vi "十八仔.vi"() -> ()   [LabVIEW 2014]
panel:
  in  "Listbox 2":i32[](listbox)
  in  "Listbox 3":i32[](listbox)
  in  "Listbox":i32[](listbox)
  in  "遊戲開始":bool
  out "總共賺取/賠掉金額":i32
  out "經歷輪數":i32
  out "此輪賺取/賠掉金額":i32
  out "賭金金額":i32
  in  "Cluster 48":T1={"Color Box 4"=16448250, "Boolean 5"=FALSE, "Boolean 11"=FALSE, "Boolean 12"=FALSE, "Boolean 13"=FALSE, "Boolean 14"=FALSE, "Boolean 15"=FALSE}
  in  "Cluster 47":T2={"Color Box 2"=16777215, "Boolean"=FALSE, "Boolean 3"=FALSE, "Boolean 2"=FALSE}
  in  "Cluster 46":T3={"Color Box"=16777215, "Boolean"=FALSE, "Boolean 2"=FALSE}
  in  "Cluster 45":T4={"Color Box"=16777215, "Boolean"=FALSE}
  in  "Cluster 44":T5={"Color Box"=16777215, "Boolean 4"=FALSE, "Boolean 5"=FALSE, "Boolean 6"=FALSE, "Boolean 7"=FALSE, "Boolean 8"=FALSE}
  in  "Cluster 43":T6={"Color Box 2"=16777215, "Boolean 3"=FALSE, "Boolean 4"=FALSE, "Boolean 6"=FALSE, "Boolean 5"=FALSE}
  in  "Cluster 42":T1={"Color Box 4"=16448250, "Boolean 5"=FALSE, "Boolean 11"=FALSE, "Boolean 12"=FALSE, "Boolean 13"=FALSE, "Boolean 14"=FALSE, "Boolean 15"=FALSE}
  in  "Cluster 41":T2={"Color Box 2"=16777215, "Boolean"=FALSE, "Boolean 3"=FALSE, "Boolean 2"=FALSE}
  in  "Cluster 40":T3={"Color Box"=16777215, "Boolean"=FALSE, "Boolean 2"=FALSE}
  in  "Cluster 39":T4={"Color Box"=16777215, "Boolean"=FALSE}
  in  "Cluster 38":T5={"Color Box"=16777215, "Boolean 4"=FALSE, "Boolean 5"=FALSE, "Boolean 6"=FALSE, "Boolean 7"=FALSE, "Boolean 8"=FALSE}
  in  "Cluster 37":T6={"Color Box 2"=16777215, "Boolean 3"=FALSE, "Boolean 4"=FALSE, "Boolean 6"=FALSE, "Boolean 5"=FALSE}
  in  "Cluster 36":T5={"Color Box"=16777215, "Boolean 4"=FALSE, "Boolean 5"=FALSE, "Boolean 6"=FALSE, "Boolean 7"=FALSE, "Boolean 8"=FALSE}
  in  "Cluster 35":T6={"Color Box 2"=16777215, "Boolean 3"=FALSE, "Boolean 4"=FALSE, "Boolean 6"=FALSE, "Boolean 5"=FALSE}
  in  "Cluster 34":T1={"Color Box 4"=16448250, "Boolean 5"=FALSE, "Boolean 11"=FALSE, "Boolean 12"=FALSE, "Boolean 13"=FALSE, "Boolean 14"=FALSE, "Boolean 15"=FALSE}
  in  "Cluster 33":T2={"Color Box 2"=16777215, "Boolean"=FALSE, "Boolean 3"=FALSE, "Boolean 2"=FALSE}
  in  "Cluster 32":T3={"Color Box"=16777215, "Boolean"=FALSE, "Boolean 2"=FALSE}
  in  "Cluster 31":T4={"Color Box"=16777215, "Boolean"=FALSE}
  in  "Cluster 30":T1={"Color Box 4"=16448250, "Boolean 5"=FALSE, "Boolean 11"=FALSE, "Boolean 12"=FALSE, "Boolean 13"=FALSE, "Boolean 14"=FALSE, "Boolean 15"=FALSE}
  in  "Cluster 29":T2={"Color Box 2"=16777215, "Boolean"=FALSE, "Boolean 3"=FALSE, "Boolean 2"=FALSE}
  in  "Cluster 28":T3={"Color Box"=16777215, "Boolean"=FALSE, "Boolean 2"=FALSE}
  in  "Cluster 27":T4={"Color Box"=16777215, "Boolean"=FALSE}
  in  "Cluster 26":T5={"Color Box"=16777215, "Boolean 4"=FALSE, "Boolean 5"=FALSE, "Boolean 6"=FALSE, "Boolean 7"=FALSE, "Boolean 8"=FALSE}
  in  "Cluster 25":T6={"Color Box 2"=16777215, "Boolean 3"=FALSE, "Boolean 4"=FALSE, "Boolean 6"=FALSE, "Boolean 5"=FALSE}
  in  "Cluster 24":T5={"Color Box"=16777215, "Boolean 4"=FALSE, "Boolean 5"=FALSE, "Boolean 6"=FALSE, "Boolean 7"=FALSE, "Boolean 8"=FALSE}
  in  "Cluster 23":T6={"Color Box 2"=16777215, "Boolean 3"=FALSE, "Boolean 4"=FALSE, "Boolean 6"=FALSE, "Boolean 5"=FALSE}
  in  "Cluster 22":T1={"Color Box 4"=16448250, "Boolean 5"=FALSE, "Boolean 11"=FALSE, "Boolean 12"=FALSE, "Boolean 13"=FALSE, "Boolean 14"=FALSE, "Boolean 15"=FALSE}
  in  "Cluster 21":T2={"Color Box 2"=16777215, "Boolean"=FALSE, "Boolean 3"=FALSE, "Boolean 2"=FALSE}
  in  "Cluster 20":T3={"Color Box"=16777215, "Boolean"=FALSE, "Boolean 2"=FALSE}
  in  "Cluster 19":T4={"Color Box"=16777215, "Boolean"=FALSE}
  in  "Cluster 18":T3={"Color Box"=16777215, "Boolean"=FALSE, "Boolean 2"=FALSE}
  in  "Cluster 17":T4={"Color Box"=16777215, "Boolean"=FALSE}
  in  "Cluster 16":T5={"Color Box"=16777215, "Boolean 4"=FALSE, "Boolean 5"=FALSE, "Boolean 6"=FALSE, "Boolean 7"=FALSE, "Boolean 8"=FALSE}
  in  "Cluster 15":T6={"Color Box 2"=16777215, "Boolean 3"=FALSE, "Boolean 4"=FALSE, "Boolean 6"=FALSE, "Boolean 5"=FALSE}
  in  "Cluster 14":T1={"Color Box 4"=16448250, "Boolean 5"=FALSE, "Boolean 11"=FALSE, "Boolean 12"=FALSE, "Boolean 13"=FALSE, "Boolean 14"=FALSE, "Boolean 15"=FALSE}
  in  "Cluster 13":T2={"Color Box 2"=16777215, "Boolean"=FALSE, "Boolean 3"=FALSE, "Boolean 2"=FALSE}
  in  "Cluster 12":T5={"Color Box"=16777215, "Boolean 4"=FALSE, "Boolean 5"=FALSE, "Boolean 6"=FALSE, "Boolean 7"=FALSE, "Boolean 8"=FALSE}
  in  "Cluster 11":T6={"Color Box 2"=16777215, "Boolean 3"=FALSE, "Boolean 4"=FALSE, "Boolean 6"=FALSE, "Boolean 5"=FALSE}
  in  "Cluster 10":T1={"Color Box 4"=16448250, "Boolean 5"=FALSE, "Boolean 11"=FALSE, "Boolean 12"=FALSE, "Boolean 13"=FALSE, "Boolean 14"=FALSE, "Boolean 15"=FALSE}
  in  "Cluster 9":T2={"Color Box 2"=16777215, "Boolean"=FALSE, "Boolean 3"=FALSE, "Boolean 2"=FALSE}
  in  "Cluster 8":T3={"Color Box"=16777215, "Boolean"=FALSE, "Boolean 2"=FALSE}
  in  "Cluster 7":T4={"Color Box"=16777215, "Boolean"=FALSE}
  in  "Cluster 4":T6={"Color Box 2"=16777215, "Boolean 3"=FALSE, "Boolean 4"=FALSE, "Boolean 6"=FALSE, "Boolean 5"=FALSE}
  in  "Cluster 6":T1={"Color Box 4"=16448250, "Boolean 5"=FALSE, "Boolean 11"=FALSE, "Boolean 12"=FALSE, "Boolean 13"=FALSE, "Boolean 14"=FALSE, "Boolean 15"=FALSE}
  in  "Cluster 3":T2={"Color Box 2"=16777215, "Boolean"=FALSE, "Boolean 3"=FALSE, "Boolean 2"=FALSE}
  in  "Cluster 2":T3={"Color Box"=16777215, "Boolean"=FALSE, "Boolean 2"=FALSE}
  in  "Cluster":T4={"Color Box"=16777215, "Boolean"=FALSE}
  in  "Cluster 5":T5={"Color Box"=16777215, "Boolean 4"=FALSE, "Boolean 5"=FALSE, "Boolean 6"=FALSE, "Boolean 7"=FALSE, "Boolean 8"=FALSE}
  out "Enum":enum16{"otherside", "myside"}(ring)
  in  "停止擲骰子":bool
  out "玩家計算點數之兩顆骰子":i32[](array[numeric])
  out "莊家計算點數之兩顆骰子":i32[](array[numeric])
  out "玩家是否是一色":bool
  out "莊家是否是一色":bool
  out "玩家所得點數":i32
  out "莊家所得點數":i32
  in  "退出遊戲":bool
  in  "進入下一輪":bool
  out "玩家重複累加器":i32
  out "玩家骰子點數":i32[](array[numeric])
  in  "下注金額":i32=10 min=10 max=30
  in  "賠率":i32=3 min=3 max=8
  out "莊家重複累加器":i32
  out "莊家骰子點數":i32[](array[numeric])
  # "遊戲介紹:"
  # "遊戲操作:"
  # "注意事項:"
  # "以上說明都看完沒問題的話，\n就可以按下遊戲開始開始遊玩囉!\n                        ↓"
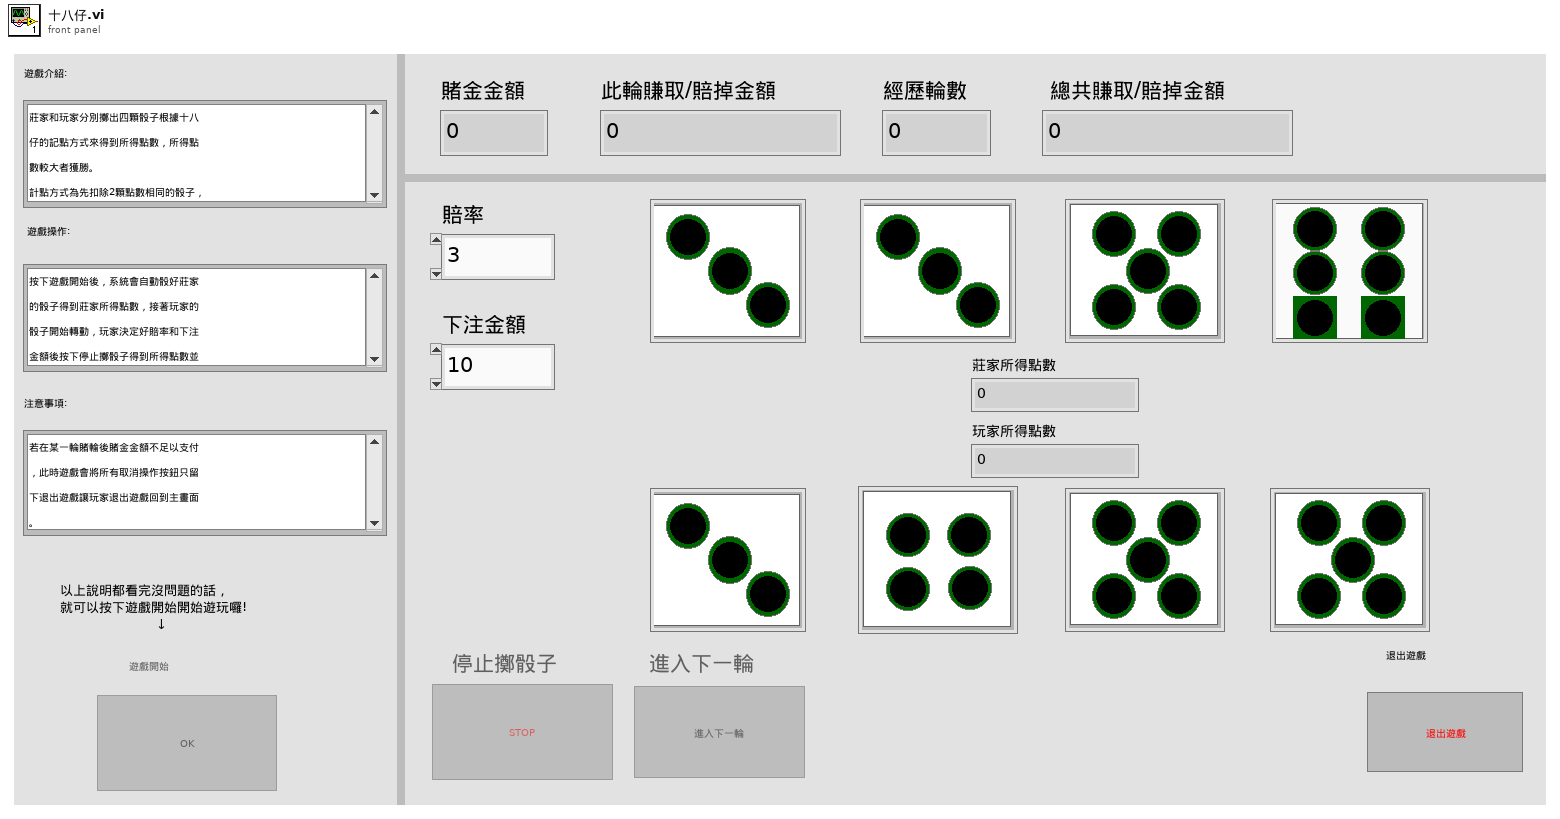
[diagram p1: front panel]
types:
  T1 = typedef "點數六.ctl" = cluster{"Color Box 4":u32, "Boolean 5":bool, "Boolean 11":bool, "Boolean 12":bool, "Boolean 13":bool, "Boolean 14":bool, "Boolean 15":bool}
  T2 = typedef "點數三.ctl" = cluster{"Color Box 2":u32, "Boolean":bool, "Boolean 3":bool, "Boolean 2":bool}
  T3 = typedef "點數二.ctl" = cluster{"Color Box":u32, "Boolean":bool, "Boolean 2":bool}
  T4 = typedef "點數一.ctl" = cluster{"Color Box":u32, "Boolean":bool}
  T5 = typedef "き.ctl" = cluster{"Color Box":u32, "Boolean 4":bool, "Boolean 5":bool, "Boolean 6":bool, "Boolean 7":bool, "Boolean 8":bool}
  T6 = typedef "點數四.ctl" = cluster{"Color Box 2":u32, "Boolean 3":bool, "Boolean 4":bool, "Boolean 6":bool, "Boolean 5":bool}
  T7 = enum16{"wait start button press", "restart", "compare and jude win or lose", "my side jude and display result", "my side throw dice and arrangement", "other side jude and display result", "other side throw dice and arrangement", "init"}
  T8 = enum8{"Enabled", "Disabled", "Disabled and Grayed Out"}
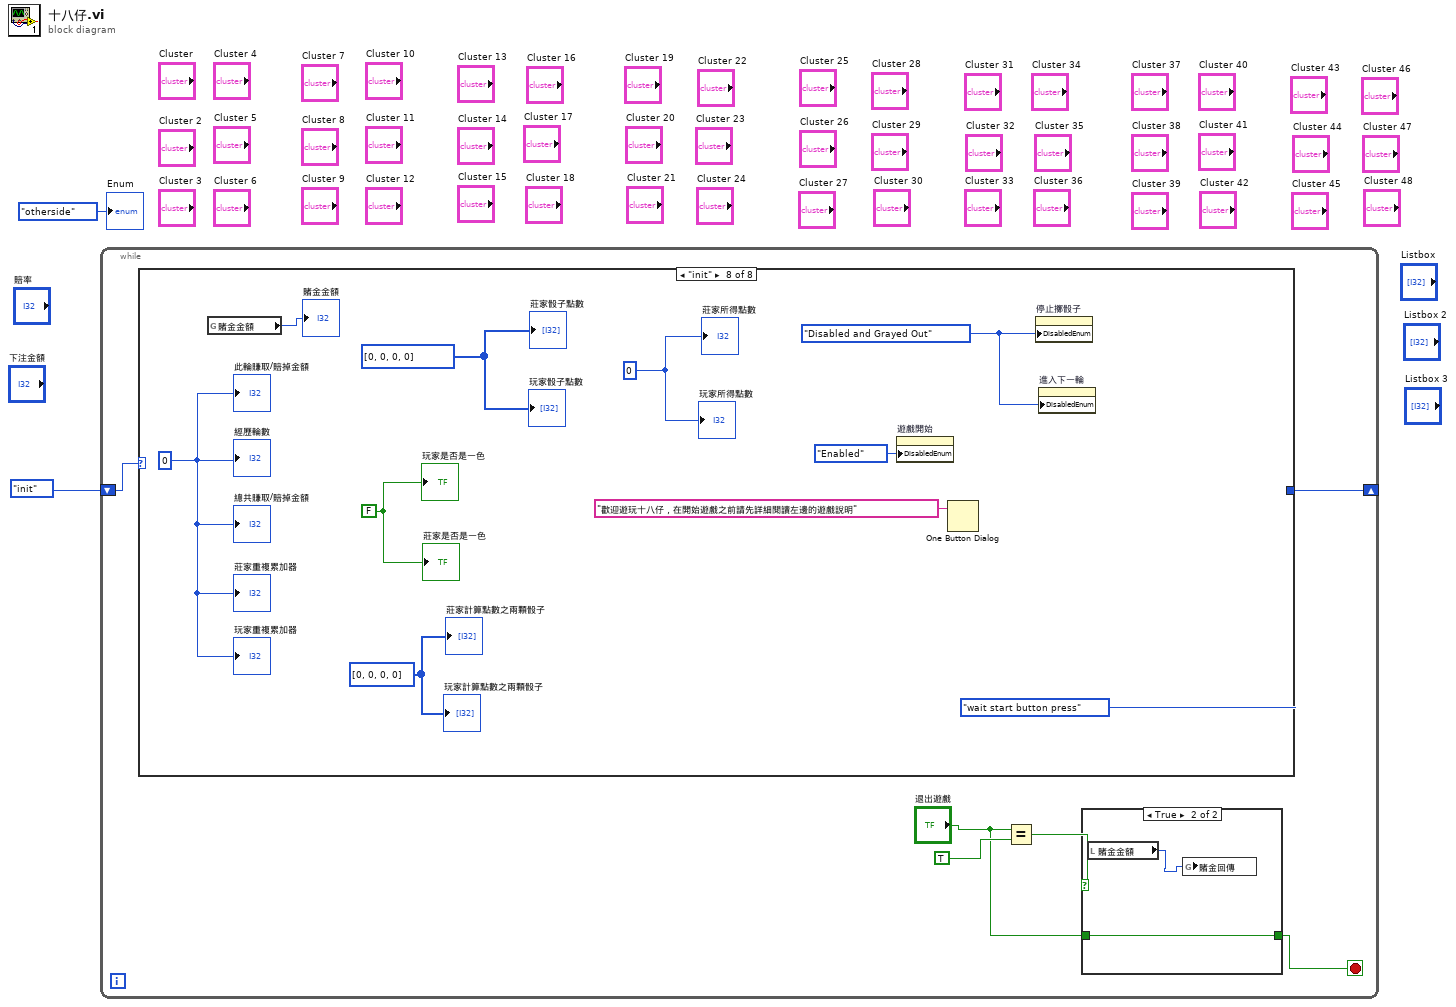
[diagram p0: block diagram]
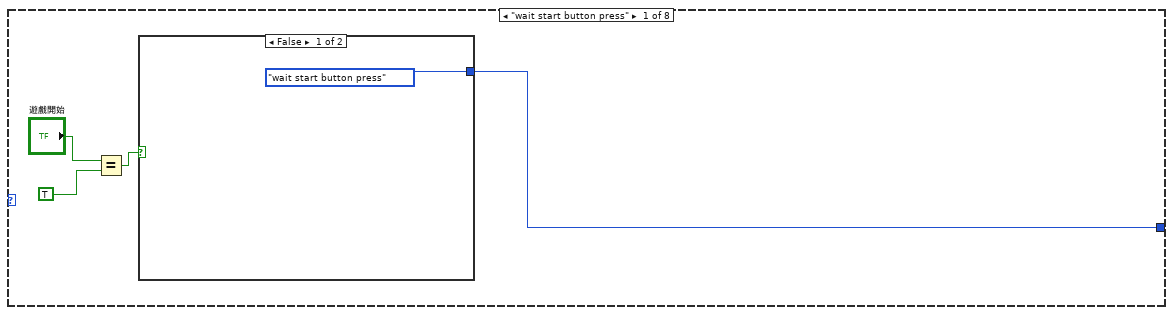
[diagram p3: hidden frame]
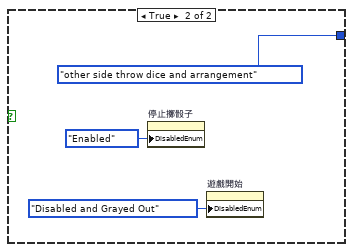
[diagram p4: hidden frame]
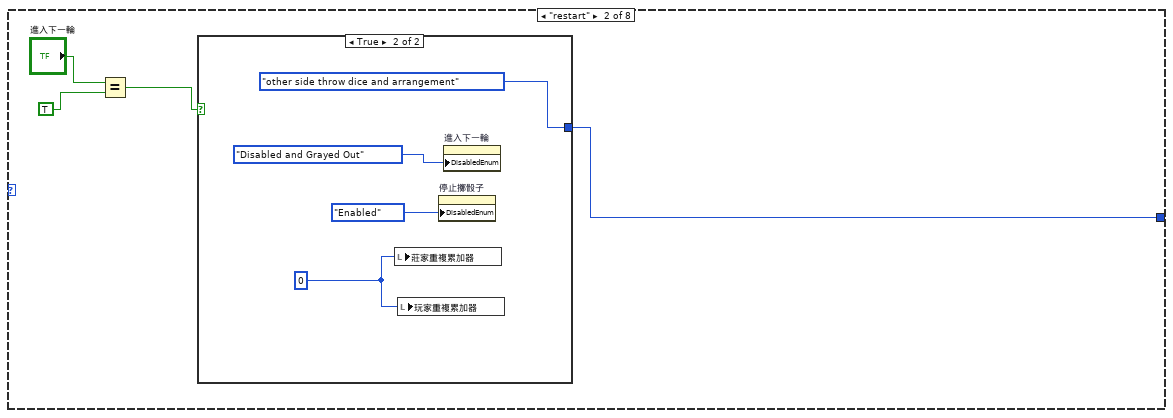
[diagram p5: hidden frame]
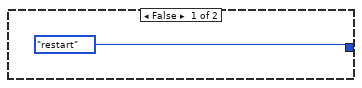
[diagram p6: hidden frame]
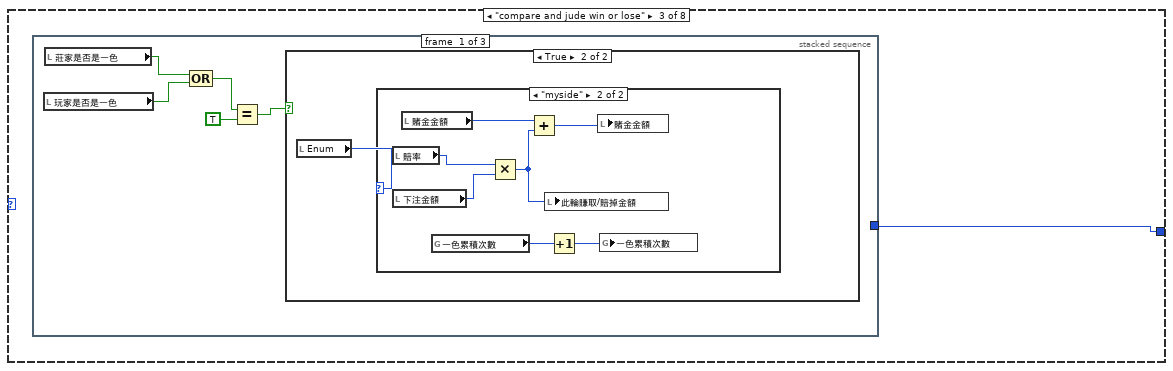
[diagram p7: hidden frame]
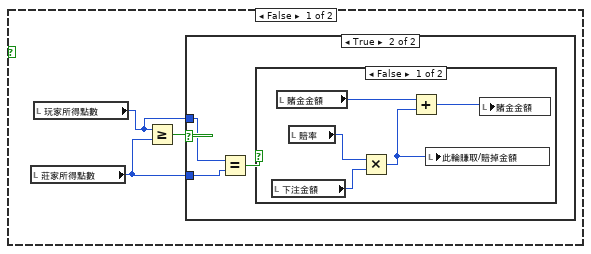
[diagram p8: hidden frame]
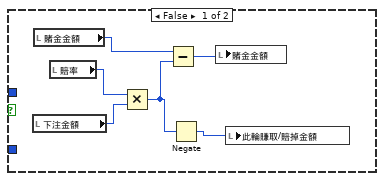
[diagram p9: hidden frame]
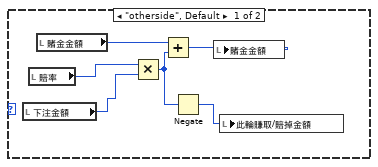
[diagram p11: hidden frame]
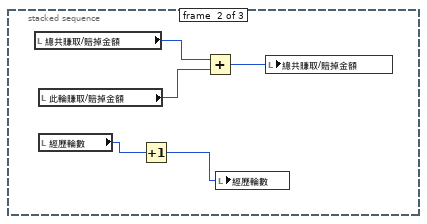
[diagram p12: hidden frame]
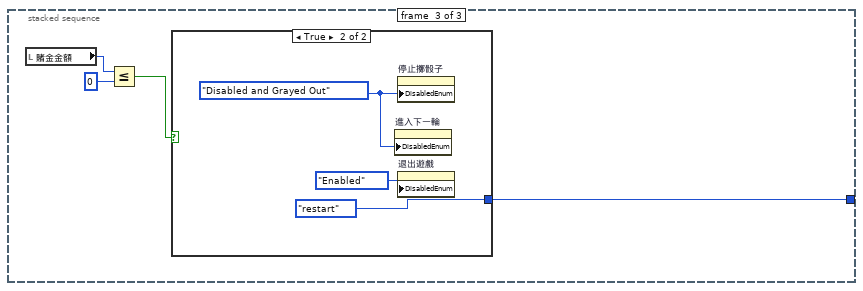
[diagram p13: hidden frame]
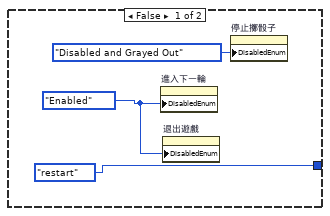
[diagram p14: hidden frame]
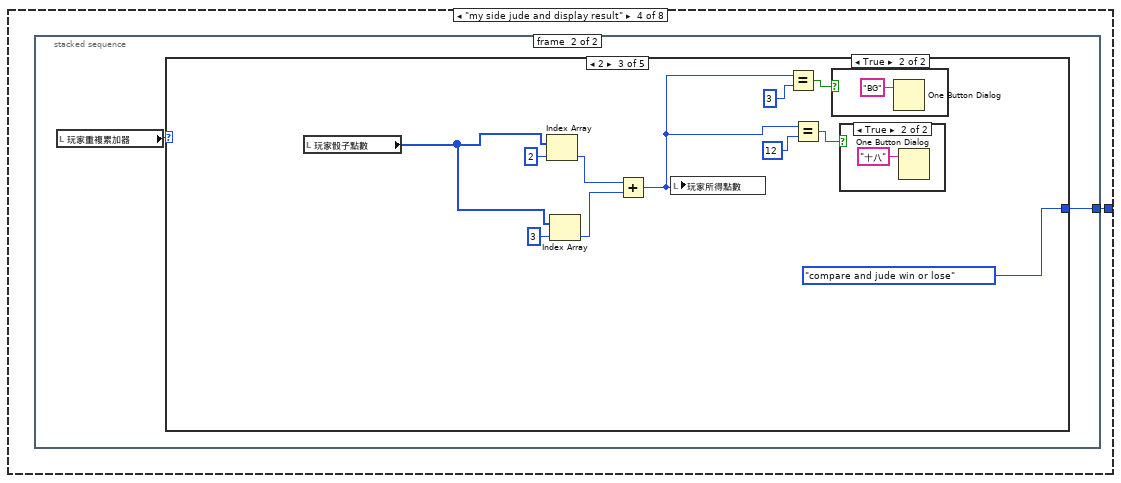
[diagram p15: hidden frame]
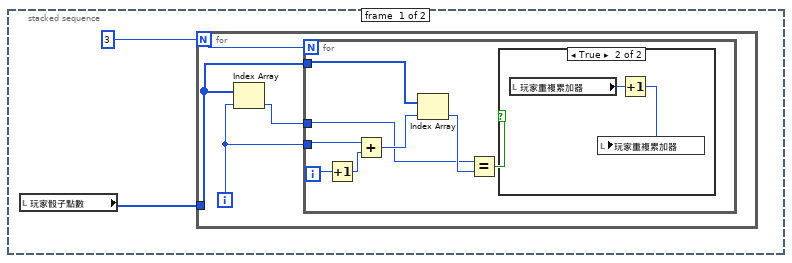
[diagram p16: hidden frame]
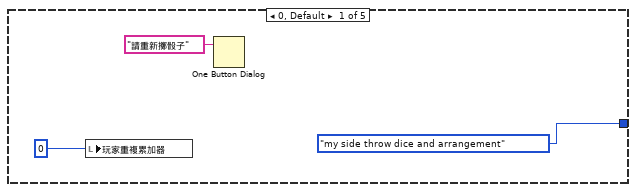
[diagram p18: hidden frame]
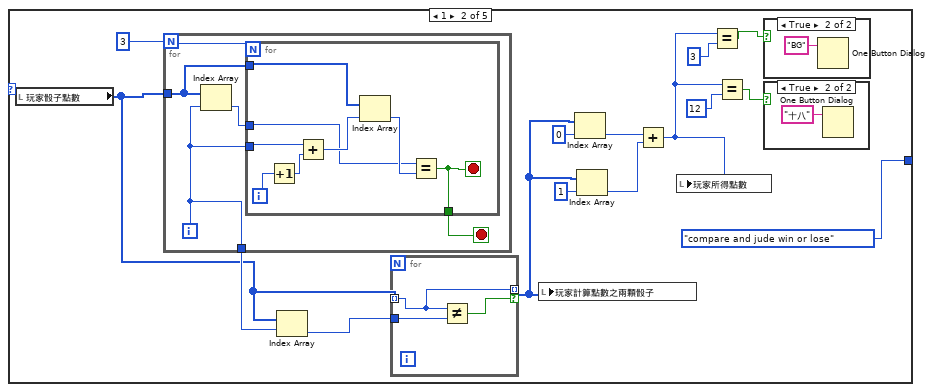
[diagram p19: hidden frame]
diagram:
  n1 = while {
    shift-right: [w7] -> _
    shift-left: T7."init" -> [w8]
    stop <- w4 stop-if-true
    n2 = case shown="\"init\"" w8 {
      tunnel: [w12 w20 w29 w81 T7."my side jude and display result" w225 T7."other side jude and display result" T7."wait start button press"] -> w7
      frame "wait start button press" {
        n3 = Equal?(x="遊戲開始", y=TRUE) -> (x = y?=w13:bool)
        n4 = case shown="False" w13 {
          tunnel: [T7."wait start button press" T7."other side throw dice and arrangement"] -> w12
          frame False {
          }
          frame True {
            n5 = property on="停止擲骰子" class="Bool"("DisabledEnum"=T8."Enabled" ("Disabled")) -> ()  [unwired: 2 in, 2 out]
            n6 = property on="遊戲開始" class="Bool"("DisabledEnum"=T8."Disabled and Grayed Out" ("Disabled")) -> ()  [unwired: 2 in, 2 out]
          }
        }
      }
      frame "restart" {
        n7 = Equal?(x="進入下一輪", y=TRUE) -> (x = y?=w21:bool)
        n8 = case shown="True" w21 {
          tunnel: [T7."restart" T7."other side throw dice and arrangement"] -> w20
          frame False {
          }
          frame True {
            w26 = 0
            n9 = local write "莊家重複累加器"(w26) -> ()
            n10 = local write "玩家重複累加器"(w26) -> ()
            n11 = property on="停止擲骰子" class="Bool"("DisabledEnum"=T8."Enabled" ("Disabled")) -> ()  [unwired: 2 in, 2 out]
            n12 = property on="進入下一輪" class="Bool"("DisabledEnum"=T8."Disabled and Grayed Out" ("Disabled")) -> ()  [unwired: 2 in, 2 out]
          }
        }
      }
      frame "compare and jude win or lose" {
        n13 = stacked-sequence {
          tunnel: [_ _ w71] -> w29
          frame #0 {
            n14 = local read "玩家是否是一色"() -> (w33:bool)
            n15 = local read "莊家是否是一色"() -> (w34:bool)
            n16 = Compound Arithmetic op=OR(w34, w33) -> (w32:bool)
            n17 = Equal?(x=w32, y=TRUE) -> (x = y?=w30:bool)
            n18 = case shown="True" w30 {
              frame False {
                n19 = local read "莊家所得點數"() -> (w35:i32)
                n20 = local read "玩家所得點數"() -> (w36:i32)
                n21 = Greater Or Equal?(x=w36, y=w35) -> (x >= y?=w37:bool)
                n22 = case shown="True" w37 {
                  tunnel: w36 -> [_ w46]
                  tunnel: w35 -> [_ w45]
                  frame False {
                    n23 = local read "下注金額"() -> (w41:i32)
                    n24 = local read "賭金金額"() -> (w43:i32)
                    n25 = local read "賠率"() -> (w42:i32)
                    n26 = Multiply(x=w42, y=w41) -> (x*y=w39:i32)
                    n27 = Subtract(x=w43, y=w39) -> (x-y=w40:i32)
                    n28 = Negate(x=w39) -> (-x=w38:i32)
                    n29 = local write "賭金金額"(w40) -> ()
                    n30 = local write "此輪賺取/賠掉金額"(w38) -> ()
                  }
                  frame True {
                    n31 = Equal?(x=w46, y=w45) -> (x = y?=w44:bool)
                    n32 = case shown="False" w44 {
                      frame False {
                        n33 = local read "下注金額"() -> (w49:i32)
                        n34 = local read "賭金金額"() -> (w51:i32)
                        n35 = local read "賠率"() -> (w50:i32)
                        n36 = Multiply(x=w50, y=w49) -> (x*y=w47:i32)
                        n37 = Add(x=w51, y=w47) -> (x+y=w48:i32)
                        n38 = local write "此輪賺取/賠掉金額"(w47) -> ()
                        n39 = local write "賭金金額"(w48) -> ()
                      }
                      frame True {
                      }
                    }
                  }
                }
              }
              frame True {
                n40 = local read "Enum"() -> (w52:enum16{"otherside", "myside"})
                n41 = case shown="\"myside\"" w52 {
                  frame "otherside", Default {
                    n42 = local read "下注金額"() -> (w58:i32)
                    n43 = local read "賠率"() -> (w57:i32)
                    n44 = local read "賭金金額"() -> (w56:i32)
                    n45 = Multiply(x=w57, y=w58) -> (x*y=w53:i32)
                    n46 = Add(x=w56, y=w53) -> (x+y=w55:i32)
                    n47 = Negate(x=w53) -> (-x=w54:i32)
                    n48 = local write "賭金金額"(w55) -> ()
                    n49 = local write "此輪賺取/賠掉金額"(w54) -> ()
                  }
                  frame "myside" {
                    n50 = local read "賠率"() -> (w65:i32)
                    n51 = local read "下注金額"() -> (w64:i32)
                    n52 = local read "賭金金額"() -> (w63:i32)
                    n53 = global read "global variable-一色累積次數.vi" "一色累積次數"() -> (w59:i32)
                    n54 = Multiply(x=w65, y=w64) -> (x*y=w61:i32)
                    n55 = Add(x=w63, y=w61) -> (x+y=w62:i32)
                    n56 = local write "此輪賺取/賠掉金額"(w61) -> ()
                    n57 = Increment(x=w59) -> (x+1=w60:i32)
                    n58 = local write "賭金金額"(w62) -> ()
                    n59 = global write "global variable-一色累積次數.vi" "一色累積次數"(w60) -> ()
                  }
                }
              }
            }
          }
          frame #1 {
            n60 = local read "總共賺取/賠掉金額"() -> (w70:i32)
            n61 = local read "此輪賺取/賠掉金額"() -> (w69:i32)
            n62 = local read "經歷輪數"() -> (w67:i32)
            n63 = Increment(x=w67) -> (x+1=w66:i32)
            n64 = Add(x=w70, y=w69) -> (x+y=w68:i32)
            n65 = local write "經歷輪數"(w66) -> ()
            n66 = local write "總共賺取/賠掉金額"(w68) -> ()
          }
          frame #2 {
            n67 = local read "賭金金額"() -> (w74:i32)
            n68 = Less Or Equal?(x=w74, y=0) -> (x <= y?=w72:bool)
            n69 = case shown="True" w72 {
              tunnel: [T7."restart" T7."restart"] -> w71
              frame False {
                w75 = T8."Enabled" ("Disabled")
                n70 = property on="進入下一輪" class="Bool"("DisabledEnum"=w75) -> ()  [unwired: 2 in, 2 out]
                n71 = property on="退出遊戲" class="Bool"("DisabledEnum"=w75) -> ()  [unwired: 2 in, 2 out]
                n72 = property on="停止擲骰子" class="Bool"("DisabledEnum"=T8."Disabled and Grayed Out" ("Disabled")) -> ()  [unwired: 2 in, 2 out]
              }
              frame True {
                w80 = T8."Disabled and Grayed Out" ("Disabled")
                n73 = property on="進入下一輪" class="Bool"("DisabledEnum"=w80) -> ()  [unwired: 2 in, 2 out]
                n74 = property on="停止擲骰子" class="Bool"("DisabledEnum"=w80) -> ()  [unwired: 2 in, 2 out]
                n75 = property on="退出遊戲" class="Bool"("DisabledEnum"=T8."Enabled" ("Disabled")) -> ()  [unwired: 2 in, 2 out]
              }
            }
          }
        }
      }
      frame "my side jude and display result" {
        n76 = stacked-sequence {
          tunnel: [_ w98] -> w81
          frame #0 {
            n77 = local read "玩家骰子點數"() -> (w83:i32[])
            n78 = for {
              N: 3 -> [w85]
              tunnel: w83 -> [w84]
              i -> [w87]
              n79 = Index Array(array=w84, index=w87) -> (element=w86:i32)
              n80 = for {
                N: w85 -> [_]
                tunnel: w87 -> [w93]
                tunnel: w84 -> [w91]
                tunnel: w86 -> [w89]
                i -> [w95]
                n81 = Increment(x=w95) -> (x+1=w94:i32)
                n82 = Add(x=w93, y=w94) -> (x+y=w92:i32)
                n83 = Index Array(array=w91, index=w92) -> (element=w90:i32)
                n84 = Equal?(x=w89, y=w90) -> (x = y?=w88:bool)
                n85 = case shown="True" w88 {
                  frame False {
                  }
                  frame True {
                    n86 = local read "玩家重複累加器"() -> (w97:i32)
                    n87 = Increment(x=w97) -> (x+1=w96:i32)
                    n88 = local write "玩家重複累加器"(w96) -> ()
                  }
                }
              }
            }
          }
          frame #1 {
            n89 = local read "玩家重複累加器"() -> (w99:i32)
            n90 = case shown="2" w99 {
              tunnel: [T7."my side throw dice and arrangement" T7."compare and jude win or lose" T7."compare and jude win or lose" T7."my side throw dice and arrangement" T7."compare and jude win or lose"] -> w98
              frame 0, Default {
                n91 = local write "玩家重複累加器"(0) -> ()
                n92 = One Button Dialog(message="請重新擲骰子") -> ()  [unwired: 1 in, 1 out]
              }
              frame 1 {
                n93 = local read "玩家骰子點數"() -> (w116:i32[])
                n94 = for {
                  N: 3 -> [w126]
                  tunnel: w116 -> [w125]
                  tunnel: [w123] -> w117
                  i -> [w123]
                  stop <- w124 stop-if-true
                  n95 = Index Array(array=w125, index=w123) -> (element=w127:i32)
                  n96 = for {
                    N: w126 -> [_]
                    tunnel: w123 -> [w133]
                    tunnel: w125 -> [w131]
                    tunnel: w127 -> [w129]
                    tunnel: [w128] -> w124
                    i -> [w135]
                    stop <- w128 stop-if-true
                    n97 = Increment(x=w135) -> (x+1=w134:i32)
                    n98 = Add(x=w133, y=w134) -> (x+y=w132:i32)
                    n99 = Index Array(array=w131, index=w132) -> (element=w130:i32)
                    n100 = Equal?(x=w129, y=w130) -> (x = y?=w128:bool)
                  }
                }
                n101 = Index Array(array=w116, index=w117) -> (element=w115:i32)
                n102 = for {
                  tunnel: w116 -> [w121] mode=indexing
                  tunnel: w115 -> [w122]
                  tunnel: [w121] -> w112 mode=indexing if=w120
                  n103 = Not Equal?(x=w121, y=w122) -> (x != y?=w120:bool)
                }
                n104 = local write "玩家計算點數之兩顆骰子"(w112) -> ()
                n105 = Index Array(array=w112, index=0) -> (element=w111:i32)
                n106 = Index Array(array=w112, index=1) -> (element=w110:i32)
                n107 = Add(x=w111, y=w110) -> (x+y=w107:i32)
                n108 = local write "玩家所得點數"(w107) -> ()
                n109 = Equal?(x=w107, y=3) -> (x = y?=w105:bool)
                n110 = Equal?(x=w107, y=12) -> (x = y?=w104:bool)
                n111 = case shown="True" w105 {
                  frame False {
                  }
                  frame True {
                    n112 = One Button Dialog(message="BG") -> ()  [unwired: 1 in, 1 out]
                  }
                }
                n113 = case shown="True" w104 {
                  frame False {
                  }
                  frame True {
                    n114 = One Button Dialog(message="十八") -> ()  [unwired: 1 in, 1 out]
                  }
                }
              }
              frame 2 {
                n115 = local read "玩家骰子點數"() -> (w142:i32[])
                n116 = Index Array(array=w142, index=2) -> (element=w144:i32)
                n117 = Index Array(array=w142, index=3) -> (element=w143:i32)
                n118 = Add(x=w144, y=w143) -> (x+y=w136:i32)
                n119 = local write "玩家所得點數"(w136) -> ()
                n120 = Equal?(x=w136, y=3) -> (x = y?=w137:bool)
                n121 = Equal?(x=w136, y=12) -> (x = y?=w138:bool)
                n122 = case shown="True" w137 {
                  frame False {
                  }
                  frame True {
                    n123 = One Button Dialog(message="BG") -> ()  [unwired: 1 in, 1 out]
                  }
                }
                n124 = case shown="True" w138 {
                  frame False {
                  }
                  frame True {
                    n125 = One Button Dialog(message="十八") -> ()  [unwired: 1 in, 1 out]
                  }
                }
              }
              frame 3 {
                n126 = One Button Dialog(message="請重新擲骰子") -> ()  [unwired: 1 in, 1 out]
                n127 = local write "玩家重複累加器"(0) -> ()
              }
              frame 6 {
                n128 = local write "玩家是否是一色"(TRUE) -> ()
                n129 = local write "Enum"(enum16{"otherside", "myside"}."myside") -> ()
                n130 = One Button Dialog(message="恭喜玩家骰到一色!") -> ()  [unwired: 1 in, 1 out]
              }
            }
          }
        }
      }
      frame "my side throw dice and arrangement" {
        n131 = while {
          stop <- "停止擲骰子" stop-if-true
          n132 = for {
            N: 4 -> [_]
            tunnel: [w219] -> w169 mode=indexing
            n133 = Random Number (0-1)() -> (number: 0 to 1=w224:dbl)
            n134 = Multiply(x=w224, y=6.0) -> (x*y=w222:dbl)
            n135 = Add(x=w222, y=0.5) -> (x+y=w220:dbl)
            n136 = To Long Integer(number=w220) -> (32bit integer=w219:i32)
          }
          n137 = Sort 1D Array(array=w169) -> (sorted array=w163:i32[])
          n138 = Wait Until Next ms Multiple(millisecond multiple=u32 100) -> ()  [unwired: 1 out]
          n139 = local write "玩家骰子點數"(w163) -> ()
          n140 = Index Array(array=w163, index=0) -> (element=w162:i32)
          n141 = case shown="1, Default" w162 {
            frame 1, Default {
              w207 = FALSE
              n142 = property on="Cluster 27" class="Clust (strict)"("Visible"=TRUE) -> ()  [unwired: 2 in, 2 out]
              n143 = property on="Cluster 29" class="Clust (strict)"("Visible"=w207) -> ()  [unwired: 2 in, 2 out]
              n144 = property on="Cluster 28" class="Clust (strict)"("Visible"=w207) -> ()  [unwired: 2 in, 2 out]
              n145 = property on="Cluster 26" class="Clust (strict)"("Visible"=w207) -> ()  [unwired: 2 in, 2 out]
              n146 = property on="Cluster 30" class="Clust (strict)"("Visible"=w207) -> ()  [unwired: 2 in, 2 out]
              n147 = property on="Cluster 25" class="Clust (strict)"("Visible"=w207) -> ()  [unwired: 2 in, 2 out]
            }
            frame 2 {
              w210 = FALSE
              n148 = property on="Cluster 26" class="Clust (strict)"("Visible"=w210) -> ()  [unwired: 2 in, 2 out]
              n149 = property on="Cluster 27" class="Clust (strict)"("Visible"=w210) -> ()  [unwired: 2 in, 2 out]
              n150 = property on="Cluster 25" class="Clust (strict)"("Visible"=w210) -> ()  [unwired: 2 in, 2 out]
              n151 = property on="Cluster 28" class="Clust (strict)"("Visible"=TRUE) -> ()  [unwired: 2 in, 2 out]
              n152 = property on="Cluster 29" class="Clust (strict)"("Visible"=w210) -> ()  [unwired: 2 in, 2 out]
              n153 = property on="Cluster 30" class="Clust (strict)"("Visible"=w210) -> ()  [unwired: 2 in, 2 out]
            }
            frame 3 {
              w212 = FALSE
              n154 = property on="Cluster 28" class="Clust (strict)"("Visible"=w212) -> ()  [unwired: 2 in, 2 out]
              n155 = property on="Cluster 26" class="Clust (strict)"("Visible"=w212) -> ()  [unwired: 2 in, 2 out]
              n156 = property on="Cluster 25" class="Clust (strict)"("Visible"=w212) -> ()  [unwired: 2 in, 2 out]
              n157 = property on="Cluster 29" class="Clust (strict)"("Visible"=TRUE) -> ()  [unwired: 2 in, 2 out]
              n158 = property on="Cluster 27" class="Clust (strict)"("Visible"=w212) -> ()  [unwired: 2 in, 2 out]
              n159 = property on="Cluster 30" class="Clust (strict)"("Visible"=w212) -> ()  [unwired: 2 in, 2 out]
            }
            frame 4 {
              w214 = FALSE
              n160 = property on="Cluster 28" class="Clust (strict)"("Visible"=w214) -> ()  [unwired: 2 in, 2 out]
              n161 = property on="Cluster 27" class="Clust (strict)"("Visible"=w214) -> ()  [unwired: 2 in, 2 out]
              n162 = property on="Cluster 26" class="Clust (strict)"("Visible"=w214) -> ()  [unwired: 2 in, 2 out]
              n163 = property on="Cluster 25" class="Clust (strict)"("Visible"=TRUE) -> ()  [unwired: 2 in, 2 out]
              n164 = property on="Cluster 29" class="Clust (strict)"("Visible"=w214) -> ()  [unwired: 2 in, 2 out]
              n165 = property on="Cluster 30" class="Clust (strict)"("Visible"=w214) -> ()  [unwired: 2 in, 2 out]
            }
            frame 5 {
              w216 = FALSE
              n166 = property on="Cluster 26" class="Clust (strict)"("Visible"=TRUE) -> ()  [unwired: 2 in, 2 out]
              n167 = property on="Cluster 27" class="Clust (strict)"("Visible"=w216) -> ()  [unwired: 2 in, 2 out]
              n168 = property on="Cluster 28" class="Clust (strict)"("Visible"=w216) -> ()  [unwired: 2 in, 2 out]
              n169 = property on="Cluster 29" class="Clust (strict)"("Visible"=w216) -> ()  [unwired: 2 in, 2 out]
              n170 = property on="Cluster 25" class="Clust (strict)"("Visible"=w216) -> ()  [unwired: 2 in, 2 out]
              n171 = property on="Cluster 30" class="Clust (strict)"("Visible"=w216) -> ()  [unwired: 2 in, 2 out]
            }
            frame 6 {
              w217 = FALSE
              n172 = property on="Cluster 27" class="Clust (strict)"("Visible"=w217) -> ()  [unwired: 2 in, 2 out]
              n173 = property on="Cluster 28" class="Clust (strict)"("Visible"=w217) -> ()  [unwired: 2 in, 2 out]
              n174 = property on="Cluster 30" class="Clust (strict)"("Visible"=TRUE) -> ()  [unwired: 2 in, 2 out]
              n175 = property on="Cluster 26" class="Clust (strict)"("Visible"=w217) -> ()  [unwired: 2 in, 2 out]
              n176 = property on="Cluster 25" class="Clust (strict)"("Visible"=w217) -> ()  [unwired: 2 in, 2 out]
              n177 = property on="Cluster 29" class="Clust (strict)"("Visible"=w217) -> ()  [unwired: 2 in, 2 out]
            }
          }
          n178 = Index Array(array=w163, index=1) -> (element=w161:i32)
          n179 = case shown="6" w161 {
            frame 1, Default {
              w195 = FALSE
              n180 = property on="Cluster 32" class="Clust (strict)"("Visible"=w195) -> ()  [unwired: 2 in, 2 out]
              n181 = property on="Cluster 34" class="Clust (strict)"("Visible"=w195) -> ()  [unwired: 2 in, 2 out]
              n182 = property on="Cluster 31" class="Clust (strict)"("Visible"=TRUE) -> ()  [unwired: 2 in, 2 out]
              n183 = property on="Cluster 33" class="Clust (strict)"("Visible"=w195) -> ()  [unwired: 2 in, 2 out]
              n184 = property on="Cluster 36" class="Clust (strict)"("Visible"=w195) -> ()  [unwired: 2 in, 2 out]
              n185 = property on="Cluster 35" class="Clust (strict)"("Visible"=w195) -> ()  [unwired: 2 in, 2 out]
            }
            frame 2 {
              w197 = FALSE
              n186 = property on="Cluster 34" class="Clust (strict)"("Visible"=w197) -> ()  [unwired: 2 in, 2 out]
              n187 = property on="Cluster 33" class="Clust (strict)"("Visible"=w197) -> ()  [unwired: 2 in, 2 out]
              n188 = property on="Cluster 31" class="Clust (strict)"("Visible"=w197) -> ()  [unwired: 2 in, 2 out]
              n189 = property on="Cluster 32" class="Clust (strict)"("Visible"=TRUE) -> ()  [unwired: 2 in, 2 out]
              n190 = property on="Cluster 36" class="Clust (strict)"("Visible"=w197) -> ()  [unwired: 2 in, 2 out]
              n191 = property on="Cluster 35" class="Clust (strict)"("Visible"=w197) -> ()  [unwired: 2 in, 2 out]
            }
            frame 3 {
              w199 = FALSE
              n192 = property on="Cluster 32" class="Clust (strict)"("Visible"=w199) -> ()  [unwired: 2 in, 2 out]
              n193 = property on="Cluster 34" class="Clust (strict)"("Visible"=w199) -> ()  [unwired: 2 in, 2 out]
              n194 = property on="Cluster 31" class="Clust (strict)"("Visible"=w199) -> ()  [unwired: 2 in, 2 out]
              n195 = property on="Cluster 33" class="Clust (strict)"("Visible"=TRUE) -> ()  [unwired: 2 in, 2 out]
              n196 = property on="Cluster 36" class="Clust (strict)"("Visible"=w199) -> ()  [unwired: 2 in, 2 out]
              n197 = property on="Cluster 35" class="Clust (strict)"("Visible"=w199) -> ()  [unwired: 2 in, 2 out]
            }
            frame 4 {
              w202 = FALSE
              n198 = property on="Cluster 31" class="Clust (strict)"("Visible"=w202) -> ()  [unwired: 2 in, 2 out]
              n199 = property on="Cluster 32" class="Clust (strict)"("Visible"=w202) -> ()  [unwired: 2 in, 2 out]
              n200 = property on="Cluster 33" class="Clust (strict)"("Visible"=w202) -> ()  [unwired: 2 in, 2 out]
              n201 = property on="Cluster 35" class="Clust (strict)"("Visible"=TRUE) -> ()  [unwired: 2 in, 2 out]
              n202 = property on="Cluster 36" class="Clust (strict)"("Visible"=w202) -> ()  [unwired: 2 in, 2 out]
              n203 = property on="Cluster 34" class="Clust (strict)"("Visible"=w202) -> ()  [unwired: 2 in, 2 out]
            }
            frame 5 {
              w203 = FALSE
              n204 = property on="Cluster 32" class="Clust (strict)"("Visible"=w203) -> ()  [unwired: 2 in, 2 out]
              n205 = property on="Cluster 34" class="Clust (strict)"("Visible"=w203) -> ()  [unwired: 2 in, 2 out]
              n206 = property on="Cluster 33" class="Clust (strict)"("Visible"=w203) -> ()  [unwired: 2 in, 2 out]
              n207 = property on="Cluster 36" class="Clust (strict)"("Visible"=TRUE) -> ()  [unwired: 2 in, 2 out]
              n208 = property on="Cluster 35" class="Clust (strict)"("Visible"=w203) -> ()  [unwired: 2 in, 2 out]
              n209 = property on="Cluster 31" class="Clust (strict)"("Visible"=w203) -> ()  [unwired: 2 in, 2 out]
            }
            frame 6 {
              w205 = FALSE
              n210 = property on="Cluster 36" class="Clust (strict)"("Visible"=w205) -> ()  [unwired: 2 in, 2 out]
              n211 = property on="Cluster 32" class="Clust (strict)"("Visible"=w205) -> ()  [unwired: 2 in, 2 out]
              n212 = property on="Cluster 33" class="Clust (strict)"("Visible"=w205) -> ()  [unwired: 2 in, 2 out]
              n213 = property on="Cluster 34" class="Clust (strict)"("Visible"=TRUE) -> ()  [unwired: 2 in, 2 out]
              n214 = property on="Cluster 31" class="Clust (strict)"("Visible"=w205) -> ()  [unwired: 2 in, 2 out]
              n215 = property on="Cluster 35" class="Clust (strict)"("Visible"=w205) -> ()  [unwired: 2 in, 2 out]
            }
          }
          n216 = Index Array(array=w163, index=2) -> (element=w160:i32)
          n217 = Index Array(array=w163, index=3) -> (element=w159:i32)
          n218 = case shown="6" w160 {
            frame 1, Default {
              w183 = FALSE
              n219 = property on="Cluster 38" class="Clust (strict)"("Visible"=w183) -> ()  [unwired: 2 in, 2 out]
              n220 = property on="Cluster 39" class="Clust (strict)"("Visible"=TRUE) -> ()  [unwired: 2 in, 2 out]
              n221 = property on="Cluster 37" class="Clust (strict)"("Visible"=w183) -> ()  [unwired: 2 in, 2 out]
              n222 = property on="Cluster 40" class="Clust (strict)"("Visible"=w183) -> ()  [unwired: 2 in, 2 out]
              n223 = property on="Cluster 42" class="Clust (strict)"("Visible"=w183) -> ()  [unwired: 2 in, 2 out]
              n224 = property on="Cluster 41" class="Clust (strict)"("Visible"=w183) -> ()  [unwired: 2 in, 2 out]
            }
            frame 2 {
              w185 = FALSE
              n225 = property on="Cluster 39" class="Clust (strict)"("Visible"=w185) -> ()  [unwired: 2 in, 2 out]
              n226 = property on="Cluster 38" class="Clust (strict)"("Visible"=w185) -> ()  [unwired: 2 in, 2 out]
              n227 = property on="Cluster 37" class="Clust (strict)"("Visible"=w185) -> ()  [unwired: 2 in, 2 out]
              n228 = property on="Cluster 40" class="Clust (strict)"("Visible"=TRUE) -> ()  [unwired: 2 in, 2 out]
              n229 = property on="Cluster 42" class="Clust (strict)"("Visible"=w185) -> ()  [unwired: 2 in, 2 out]
              n230 = property on="Cluster 41" class="Clust (strict)"("Visible"=w185) -> ()  [unwired: 2 in, 2 out]
            }
            frame 3 {
              w187 = FALSE
              n231 = property on="Cluster 38" class="Clust (strict)"("Visible"=w187) -> ()  [unwired: 2 in, 2 out]
              n232 = property on="Cluster 40" class="Clust (strict)"("Visible"=w187) -> ()  [unwired: 2 in, 2 out]
              n233 = property on="Cluster 41" class="Clust (strict)"("Visible"=TRUE) -> ()  [unwired: 2 in, 2 out]
              n234 = property on="Cluster 37" class="Clust (strict)"("Visible"=w187) -> ()  [unwired: 2 in, 2 out]
              n235 = property on="Cluster 42" class="Clust (strict)"("Visible"=w187) -> ()  [unwired: 2 in, 2 out]
              n236 = property on="Cluster 39" class="Clust (strict)"("Visible"=w187) -> ()  [unwired: 2 in, 2 out]
            }
            frame 4 {
              w189 = FALSE
              n237 = property on="Cluster 38" class="Clust (strict)"("Visible"=w189) -> ()  [unwired: 2 in, 2 out]
              n238 = property on="Cluster 39" class="Clust (strict)"("Visible"=w189) -> ()  [unwired: 2 in, 2 out]
              n239 = property on="Cluster 37" class="Clust (strict)"("Visible"=TRUE) -> ()  [unwired: 2 in, 2 out]
              n240 = property on="Cluster 40" class="Clust (strict)"("Visible"=w189) -> ()  [unwired: 2 in, 2 out]
              n241 = property on="Cluster 42" class="Clust (strict)"("Visible"=w189) -> ()  [unwired: 2 in, 2 out]
              n242 = property on="Cluster 41" class="Clust (strict)"("Visible"=w189) -> ()  [unwired: 2 in, 2 out]
            }
            frame 5 {
              w191 = FALSE
              n243 = property on="Cluster 39" class="Clust (strict)"("Visible"=w191) -> ()  [unwired: 2 in, 2 out]
              n244 = property on="Cluster 40" class="Clust (strict)"("Visible"=w191) -> ()  [unwired: 2 in, 2 out]
              n245 = property on="Cluster 38" class="Clust (strict)"("Visible"=TRUE) -> ()  [unwired: 2 in, 2 out]
              n246 = property on="Cluster 41" class="Clust (strict)"("Visible"=w191) -> ()  [unwired: 2 in, 2 out]
              n247 = property on="Cluster 37" class="Clust (strict)"("Visible"=w191) -> ()  [unwired: 2 in, 2 out]
              n248 = property on="Cluster 42" class="Clust (strict)"("Visible"=w191) -> ()  [unwired: 2 in, 2 out]
            }
            frame 6 {
              w193 = FALSE
              n249 = property on="Cluster 38" class="Clust (strict)"("Visible"=w193) -> ()  [unwired: 2 in, 2 out]
              n250 = property on="Cluster 39" class="Clust (strict)"("Visible"=w193) -> ()  [unwired: 2 in, 2 out]
              n251 = property on="Cluster 40" class="Clust (strict)"("Visible"=w193) -> ()  [unwired: 2 in, 2 out]
              n252 = property on="Cluster 42" class="Clust (strict)"("Visible"=TRUE) -> ()  [unwired: 2 in, 2 out]
              n253 = property on="Cluster 41" class="Clust (strict)"("Visible"=w193) -> ()  [unwired: 2 in, 2 out]
              n254 = property on="Cluster 37" class="Clust (strict)"("Visible"=w193) -> ()  [unwired: 2 in, 2 out]
            }
          }
          n255 = case shown="6" w159 {
            frame 1, Default {
              w171 = FALSE
              n256 = property on="Cluster 46" class="Clust (strict)"("Visible"=w171) -> ()  [unwired: 2 in, 2 out]
              n257 = property on="Cluster 43" class="Clust (strict)"("Visible"=w171) -> ()  [unwired: 2 in, 2 out]
              n258 = property on="Cluster 44" class="Clust (strict)"("Visible"=w171) -> ()  [unwired: 2 in, 2 out]
              n259 = property on="Cluster 45" class="Clust (strict)"("Visible"=TRUE) -> ()  [unwired: 2 in, 2 out]
              n260 = property on="Cluster 48" class="Clust (strict)"("Visible"=w171) -> ()  [unwired: 2 in, 2 out]
              n261 = property on="Cluster 47" class="Clust (strict)"("Visible"=w171) -> ()  [unwired: 2 in, 2 out]
            }
            frame 2 {
              w173 = FALSE
              n262 = property on="Cluster 43" class="Clust (strict)"("Visible"=w173) -> ()  [unwired: 2 in, 2 out]
              n263 = property on="Cluster 46" class="Clust (strict)"("Visible"=TRUE) -> ()  [unwired: 2 in, 2 out]
              n264 = property on="Cluster 45" class="Clust (strict)"("Visible"=w173) -> ()  [unwired: 2 in, 2 out]
              n265 = property on="Cluster 44" class="Clust (strict)"("Visible"=w173) -> ()  [unwired: 2 in, 2 out]
              n266 = property on="Cluster 48" class="Clust (strict)"("Visible"=w173) -> ()  [unwired: 2 in, 2 out]
              n267 = property on="Cluster 47" class="Clust (strict)"("Visible"=w173) -> ()  [unwired: 2 in, 2 out]
            }
            frame 3 {
              w175 = FALSE
              n268 = property on="Cluster 46" class="Clust (strict)"("Visible"=w175) -> ()  [unwired: 2 in, 2 out]
              n269 = property on="Cluster 44" class="Clust (strict)"("Visible"=w175) -> ()  [unwired: 2 in, 2 out]
              n270 = property on="Cluster 43" class="Clust (strict)"("Visible"=w175) -> ()  [unwired: 2 in, 2 out]
              n271 = property on="Cluster 47" class="Clust (strict)"("Visible"=TRUE) -> ()  [unwired: 2 in, 2 out]
              n272 = property on="Cluster 48" class="Clust (strict)"("Visible"=w175) -> ()  [unwired: 2 in, 2 out]
              n273 = property on="Cluster 45" class="Clust (strict)"("Visible"=w175) -> ()  [unwired: 2 in, 2 out]
            }
            frame 4 {
              w177 = FALSE
              n274 = property on="Cluster 45" class="Clust (strict)"("Visible"=w177) -> ()  [unwired: 2 in, 2 out]
              n275 = property on="Cluster 46" class="Clust (strict)"("Visible"=w177) -> ()  [unwired: 2 in, 2 out]
              n276 = property on="Cluster 44" class="Clust (strict)"("Visible"=w177) -> ()  [unwired: 2 in, 2 out]
              n277 = property on="Cluster 43" class="Clust (strict)"("Visible"=TRUE) -> ()  [unwired: 2 in, 2 out]
              n278 = property on="Cluster 48" class="Clust (strict)"("Visible"=w177) -> ()  [unwired: 2 in, 2 out]
              n279 = property on="Cluster 47" class="Clust (strict)"("Visible"=w177) -> ()  [unwired: 2 in, 2 out]
            }
            frame 5 {
              w179 = FALSE
              n280 = property on="Cluster 46" class="Clust (strict)"("Visible"=w179) -> ()  [unwired: 2 in, 2 out]
              n281 = property on="Cluster 45" class="Clust (strict)"("Visible"=w179) -> ()  [unwired: 2 in, 2 out]
              n282 = property on="Cluster 47" class="Clust (strict)"("Visible"=w179) -> ()  [unwired: 2 in, 2 out]
              n283 = property on="Cluster 44" class="Clust (strict)"("Visible"=TRUE) -> ()  [unwired: 2 in, 2 out]
              n284 = property on="Cluster 48" class="Clust (strict)"("Visible"=w179) -> ()  [unwired: 2 in, 2 out]
              n285 = property on="Cluster 43" class="Clust (strict)"("Visible"=w179) -> ()  [unwired: 2 in, 2 out]
            }
            frame 6 {
              w181 = FALSE
              n286 = property on="Cluster 46" class="Clust (strict)"("Visible"=w181) -> ()  [unwired: 2 in, 2 out]
              n287 = property on="Cluster 45" class="Clust (strict)"("Visible"=w181) -> ()  [unwired: 2 in, 2 out]
              n288 = property on="Cluster 44" class="Clust (strict)"("Visible"=w181) -> ()  [unwired: 2 in, 2 out]
              n289 = property on="Cluster 48" class="Clust (strict)"("Visible"=TRUE) -> ()  [unwired: 2 in, 2 out]
              n290 = property on="Cluster 47" class="Clust (strict)"("Visible"=w181) -> ()  [unwired: 2 in, 2 out]
              n291 = property on="Cluster 43" class="Clust (strict)"("Visible"=w181) -> ()  [unwired: 2 in, 2 out]
            }
          }
        }
        n292 = property on="退出遊戲" class="Bool"("DisabledEnum"=T8."Disabled and Grayed Out" ("Disabled")) -> ()  [unwired: 2 in, 2 out]
      }
      frame "other side jude and display result" {
        n293 = stacked-sequence {
          tunnel: [_ w242] -> w225
          frame #0 {
            n294 = local read "莊家骰子點數"() -> (w227:i32[])
            n295 = for {
              N: 3 -> [w229]
              tunnel: w227 -> [w228]
              i -> [w231]
              n296 = Index Array(array=w228, index=w231) -> (element=w230:i32)
              n297 = for {
                N: w229 -> [_]
                tunnel: w231 -> [w237]
                tunnel: w228 -> [w235]
                tunnel: w230 -> [w233]
                i -> [w239]
                n298 = Increment(x=w239) -> (x+1=w238:i32)
                n299 = Add(x=w237, y=w238) -> (x+y=w236:i32)
                n300 = Index Array(array=w235, index=w236) -> (element=w234:i32)
                n301 = Equal?(x=w233, y=w234) -> (x = y?=w232:bool)
                n302 = case shown="True" w232 {
                  frame False {
                  }
                  frame True {
                    n303 = local read "莊家重複累加器"() -> (w241:i32)
                    n304 = Increment(x=w241) -> (x+1=w240:i32)
                    n305 = local write "莊家重複累加器"(w240) -> ()
                  }
                }
              }
            }
          }
          frame #1 {
            n306 = local read "莊家重複累加器"() -> (w243:i32)
            n307 = case shown="6" w243 {
              tunnel: [T7."other side throw dice and arrangement" T7."my side throw dice and arrangement" T7."my side throw dice and arrangement" T7."other side throw dice and arrangement" T7."compare and jude win or lose"] -> w242
              frame 0, Default {
                n308 = local write "莊家重複累加器"(0) -> ()
              }
              frame 1 {
                n309 = local read "莊家骰子點數"() -> (w256:i32[])
                n310 = for {
                  N: 3 -> [w264]
                  tunnel: w256 -> [w263]
                  tunnel: [w261] -> w257
                  i -> [w261]
                  stop <- w262 stop-if-true
                  n311 = Index Array(array=w263, index=w261) -> (element=w265:i32)
                  n312 = for {
                    N: w264 -> [_]
                    tunnel: w261 -> [w271]
                    tunnel: w263 -> [w269]
                    tunnel: w265 -> [w267]
                    tunnel: [w266] -> w262
                    i -> [w273]
                    stop <- w266 stop-if-true
                    n313 = Increment(x=w273) -> (x+1=w272:i32)
                    n314 = Add(x=w271, y=w272) -> (x+y=w270:i32)
                    n315 = Index Array(array=w269, index=w270) -> (element=w268:i32)
                    n316 = Equal?(x=w267, y=w268) -> (x = y?=w266:bool)
                  }
                }
                n317 = Index Array(array=w256, index=w257) -> (element=w255:i32)
                n318 = for {
                  tunnel: w256 -> [w259] mode=indexing
                  tunnel: w255 -> [w260]
                  tunnel: [w259] -> w252 mode=indexing if=w258
                  n319 = Not Equal?(x=w259, y=w260) -> (x != y?=w258:bool)
                }
                n320 = local write "莊家計算點數之兩顆骰子"(w252) -> ()
                n321 = Index Array(array=w252, index=0) -> (element=w251:i32)
                n322 = Index Array(array=w252, index=1) -> (element=w250:i32)
                n323 = Add(x=w251, y=w250) -> (x+y=w249:i32)
                n324 = local write "莊家所得點數"(w249) -> ()
                n325 = One Button Dialog(message="莊家已擲好骰子，換玩家擲骰子") -> ()  [unwired: 1 in, 1 out]
              }
              frame 2 {
                n326 = local read "莊家骰子點數"() -> (w279:i32[])
                n327 = Index Array(array=w279, index=2) -> (element=w278:i32)
                n328 = Index Array(array=w279, index=3) -> (element=w277:i32)
                n329 = Add(x=w278, y=w277) -> (x+y=w276:i32)
                n330 = local write "莊家所得點數"(w276) -> ()
                n331 = One Button Dialog(message="莊家已擲好骰子，換玩家擲骰子") -> ()  [unwired: 1 in, 1 out]
              }
              frame 3 {
                n332 = local write "莊家重複累加器"(0) -> ()
              }
              frame 6 {
                n333 = local write "Enum"(enum16{"otherside", "myside"}."otherside") -> ()
                n334 = local write "莊家是否是一色"(TRUE) -> ()
                n335 = One Button Dialog(message="莊家骰出一色!") -> ()  [unwired: 1 in, 1 out]
              }
            }
          }
        }
      }
      frame "other side throw dice and arrangement" {
        n336 = for {
          N: 4 -> [_]
          tunnel: [w348] -> w298 mode=indexing
          n337 = Random Number (0-1)() -> (number: 0 to 1=w353:dbl)
          n338 = Multiply(x=w353, y=6.0) -> (x*y=w351:dbl)
          n339 = Add(x=w351, y=0.5) -> (x+y=w349:dbl)
          n340 = To Long Integer(number=w349) -> (32bit integer=w348:i32)
        }
        n341 = Sort 1D Array(array=w298) -> (sorted array=w293:i32[])
        n342 = local write "莊家骰子點數"(w293) -> ()
        n343 = Index Array(array=w293, index=0) -> (element=w291:i32)
        n344 = case shown="6" w291 {
          frame 1, Default {
            w336 = FALSE
            n345 = property on="Cluster 4" class="Clust (strict)"("Visible"=w336) -> ()  [unwired: 2 in, 2 out]
            n346 = property on="Cluster 3" class="Clust (strict)"("Visible"=w336) -> ()  [unwired: 2 in, 2 out]
            n347 = property on="Cluster 2" class="Clust (strict)"("Visible"=w336) -> ()  [unwired: 2 in, 2 out]
            n348 = property on="Cluster" class="Clust (strict)"("Visible"=TRUE) -> ()  [unwired: 2 in, 2 out]
            n349 = property on="Cluster 5" class="Clust (strict)"("Visible"=w336) -> ()  [unwired: 2 in, 2 out]
            n350 = property on="Cluster 6" class="Clust (strict)"("Visible"=w336) -> ()  [unwired: 2 in, 2 out]
          }
          frame 2 {
            w339 = FALSE
            n351 = property on="Cluster 3" class="Clust (strict)"("Visible"=w339) -> ()  [unwired: 2 in, 2 out]
            n352 = property on="Cluster 4" class="Clust (strict)"("Visible"=w339) -> ()  [unwired: 2 in, 2 out]
            n353 = property on="Cluster 2" class="Clust (strict)"("Visible"=TRUE) -> ()  [unwired: 2 in, 2 out]
            n354 = property on="Cluster" class="Clust (strict)"("Visible"=w339) -> ()  [unwired: 2 in, 2 out]
            n355 = property on="Cluster 5" class="Clust (strict)"("Visible"=w339) -> ()  [unwired: 2 in, 2 out]
            n356 = property on="Cluster 6" class="Clust (strict)"("Visible"=w339) -> ()  [unwired: 2 in, 2 out]
          }
          frame 3 {
            w340 = FALSE
            n357 = property on="Cluster 3" class="Clust (strict)"("Visible"=TRUE) -> ()  [unwired: 2 in, 2 out]
            n358 = property on="Cluster 2" class="Clust (strict)"("Visible"=w340) -> ()  [unwired: 2 in, 2 out]
            n359 = property on="Cluster 4" class="Clust (strict)"("Visible"=w340) -> ()  [unwired: 2 in, 2 out]
            n360 = property on="Cluster" class="Clust (strict)"("Visible"=w340) -> ()  [unwired: 2 in, 2 out]
            n361 = property on="Cluster 5" class="Clust (strict)"("Visible"=w340) -> ()  [unwired: 2 in, 2 out]
            n362 = property on="Cluster 6" class="Clust (strict)"("Visible"=w340) -> ()  [unwired: 2 in, 2 out]
          }
          frame 4 {
            w342 = FALSE
            n363 = property on="Cluster 2" class="Clust (strict)"("Visible"=w342) -> ()  [unwired: 2 in, 2 out]
            n364 = property on="Cluster 3" class="Clust (strict)"("Visible"=w342) -> ()  [unwired: 2 in, 2 out]
            n365 = property on="Cluster 4" class="Clust (strict)"("Visible"=TRUE) -> ()  [unwired: 2 in, 2 out]
            n366 = property on="Cluster" class="Clust (strict)"("Visible"=w342) -> ()  [unwired: 2 in, 2 out]
            n367 = property on="Cluster 5" class="Clust (strict)"("Visible"=w342) -> ()  [unwired: 2 in, 2 out]
            n368 = property on="Cluster 6" class="Clust (strict)"("Visible"=w342) -> ()  [unwired: 2 in, 2 out]
          }
          frame 5 {
            w345 = FALSE
            n369 = property on="Cluster 2" class="Clust (strict)"("Visible"=w345) -> ()  [unwired: 2 in, 2 out]
            n370 = property on="Cluster 3" class="Clust (strict)"("Visible"=w345) -> ()  [unwired: 2 in, 2 out]
            n371 = property on="Cluster 4" class="Clust (strict)"("Visible"=w345) -> ()  [unwired: 2 in, 2 out]
            n372 = property on="Cluster 5" class="Clust (strict)"("Visible"=TRUE) -> ()  [unwired: 2 in, 2 out]
            n373 = property on="Cluster 6" class="Clust (strict)"("Visible"=w345) -> ()  [unwired: 2 in, 2 out]
            n374 = property on="Cluster" class="Clust (strict)"("Visible"=w345) -> ()  [unwired: 2 in, 2 out]
          }
          frame 6 {
            w347 = FALSE
            n375 = property on="Cluster 2" class="Clust (strict)"("Visible"=w347) -> ()  [unwired: 2 in, 2 out]
            n376 = property on="Cluster 3" class="Clust (strict)"("Visible"=w347) -> ()  [unwired: 2 in, 2 out]
            n377 = property on="Cluster 4" class="Clust (strict)"("Visible"=w347) -> ()  [unwired: 2 in, 2 out]
            n378 = property on="Cluster 6" class="Clust (strict)"("Visible"=TRUE) -> ()  [unwired: 2 in, 2 out]
            n379 = property on="Cluster 5" class="Clust (strict)"("Visible"=w347) -> ()  [unwired: 2 in, 2 out]
            n380 = property on="Cluster" class="Clust (strict)"("Visible"=w347) -> ()  [unwired: 2 in, 2 out]
          }
        }
        n381 = Index Array(array=w293, index=1) -> (element=w290:i32)
        n382 = case shown="6" w290 {
          frame 1, Default {
            w324 = FALSE
            n383 = property on="Cluster 9" class="Clust (strict)"("Visible"=w324) -> ()  [unwired: 2 in, 2 out]
            n384 = property on="Cluster 8" class="Clust (strict)"("Visible"=w324) -> ()  [unwired: 2 in, 2 out]
            n385 = property on="Cluster 10" class="Clust (strict)"("Visible"=w324) -> ()  [unwired: 2 in, 2 out]
            n386 = property on="Cluster 7" class="Clust (strict)"("Visible"=TRUE) -> ()  [unwired: 2 in, 2 out]
            n387 = property on="Cluster 11" class="Clust (strict)"("Visible"=w324) -> ()  [unwired: 2 in, 2 out]
            n388 = property on="Cluster 12" class="Clust (strict)"("Visible"=w324) -> ()  [unwired: 2 in, 2 out]
          }
          frame 2 {
            w326 = FALSE
            n389 = property on="Cluster 9" class="Clust (strict)"("Visible"=w326) -> ()  [unwired: 2 in, 2 out]
            n390 = property on="Cluster 10" class="Clust (strict)"("Visible"=w326) -> ()  [unwired: 2 in, 2 out]
            n391 = property on="Cluster 7" class="Clust (strict)"("Visible"=w326) -> ()  [unwired: 2 in, 2 out]
            n392 = property on="Cluster 8" class="Clust (strict)"("Visible"=TRUE) -> ()  [unwired: 2 in, 2 out]
            n393 = property on="Cluster 11" class="Clust (strict)"("Visible"=w326) -> ()  [unwired: 2 in, 2 out]
            n394 = property on="Cluster 12" class="Clust (strict)"("Visible"=w326) -> ()  [unwired: 2 in, 2 out]
          }
          frame 3 {
            w328 = FALSE
            n395 = property on="Cluster 8" class="Clust (strict)"("Visible"=w328) -> ()  [unwired: 2 in, 2 out]
            n396 = property on="Cluster 10" class="Clust (strict)"("Visible"=w328) -> ()  [unwired: 2 in, 2 out]
            n397 = property on="Cluster 9" class="Clust (strict)"("Visible"=TRUE) -> ()  [unwired: 2 in, 2 out]
            n398 = property on="Cluster 7" class="Clust (strict)"("Visible"=w328) -> ()  [unwired: 2 in, 2 out]
            n399 = property on="Cluster 11" class="Clust (strict)"("Visible"=w328) -> ()  [unwired: 2 in, 2 out]
            n400 = property on="Cluster 12" class="Clust (strict)"("Visible"=w328) -> ()  [unwired: 2 in, 2 out]
          }
          frame 4 {
            w330 = FALSE
            n401 = property on="Cluster 7" class="Clust (strict)"("Visible"=w330) -> ()  [unwired: 2 in, 2 out]
            n402 = property on="Cluster 9" class="Clust (strict)"("Visible"=w330) -> ()  [unwired: 2 in, 2 out]
            n403 = property on="Cluster 8" class="Clust (strict)"("Visible"=w330) -> ()  [unwired: 2 in, 2 out]
            n404 = property on="Cluster 11" class="Clust (strict)"("Visible"=TRUE) -> ()  [unwired: 2 in, 2 out]
            n405 = property on="Cluster 12" class="Clust (strict)"("Visible"=w330) -> ()  [unwired: 2 in, 2 out]
            n406 = property on="Cluster 10" class="Clust (strict)"("Visible"=w330) -> ()  [unwired: 2 in, 2 out]
          }
          frame 5 {
            w332 = FALSE
            n407 = property on="Cluster 9" class="Clust (strict)"("Visible"=w332) -> ()  [unwired: 2 in, 2 out]
            n408 = property on="Cluster 8" class="Clust (strict)"("Visible"=w332) -> ()  [unwired: 2 in, 2 out]
            n409 = property on="Cluster 10" class="Clust (strict)"("Visible"=w332) -> ()  [unwired: 2 in, 2 out]
            n410 = property on="Cluster 12" class="Clust (strict)"("Visible"=TRUE) -> ()  [unwired: 2 in, 2 out]
            n411 = property on="Cluster 11" class="Clust (strict)"("Visible"=w332) -> ()  [unwired: 2 in, 2 out]
            n412 = property on="Cluster 7" class="Clust (strict)"("Visible"=w332) -> ()  [unwired: 2 in, 2 out]
          }
          frame 6 {
            w335 = FALSE
            n413 = property on="Cluster 9" class="Clust (strict)"("Visible"=w335) -> ()  [unwired: 2 in, 2 out]
            n414 = property on="Cluster 8" class="Clust (strict)"("Visible"=w335) -> ()  [unwired: 2 in, 2 out]
            n415 = property on="Cluster 12" class="Clust (strict)"("Visible"=w335) -> ()  [unwired: 2 in, 2 out]
            n416 = property on="Cluster 10" class="Clust (strict)"("Visible"=TRUE) -> ()  [unwired: 2 in, 2 out]
            n417 = property on="Cluster 7" class="Clust (strict)"("Visible"=w335) -> ()  [unwired: 2 in, 2 out]
            n418 = property on="Cluster 11" class="Clust (strict)"("Visible"=w335) -> ()  [unwired: 2 in, 2 out]
          }
        }
        n419 = Index Array(array=w293, index=2) -> (element=w289:i32)
        n420 = Index Array(array=w293, index=3) -> (element=w288:i32)
        n421 = case shown="6" w289 {
          frame 1, Default {
            w312 = FALSE
            n422 = property on="Cluster 17" class="Clust (strict)"("Visible"=TRUE) -> ()  [unwired: 2 in, 2 out]
            n423 = property on="Cluster 15" class="Clust (strict)"("Visible"=w312) -> ()  [unwired: 2 in, 2 out]
            n424 = property on="Cluster 14" class="Clust (strict)"("Visible"=w312) -> ()  [unwired: 2 in, 2 out]
            n425 = property on="Cluster 16" class="Clust (strict)"("Visible"=w312) -> ()  [unwired: 2 in, 2 out]
            n426 = property on="Cluster 18" class="Clust (strict)"("Visible"=w312) -> ()  [unwired: 2 in, 2 out]
            n427 = property on="Cluster 13" class="Clust (strict)"("Visible"=w312) -> ()  [unwired: 2 in, 2 out]
          }
          frame 2 {
            w314 = FALSE
            n428 = property on="Cluster 15" class="Clust (strict)"("Visible"=w314) -> ()  [unwired: 2 in, 2 out]
            n429 = property on="Cluster 16" class="Clust (strict)"("Visible"=w314) -> ()  [unwired: 2 in, 2 out]
            n430 = property on="Cluster 13" class="Clust (strict)"("Visible"=w314) -> ()  [unwired: 2 in, 2 out]
            n431 = property on="Cluster 18" class="Clust (strict)"("Visible"=TRUE) -> ()  [unwired: 2 in, 2 out]
            n432 = property on="Cluster 17" class="Clust (strict)"("Visible"=w314) -> ()  [unwired: 2 in, 2 out]
            n433 = property on="Cluster 14" class="Clust (strict)"("Visible"=w314) -> ()  [unwired: 2 in, 2 out]
          }
          frame 3 {
            w316 = FALSE
            n434 = property on="Cluster 14" class="Clust (strict)"("Visible"=w316) -> ()  [unwired: 2 in, 2 out]
            n435 = property on="Cluster 16" class="Clust (strict)"("Visible"=w316) -> ()  [unwired: 2 in, 2 out]
            n436 = property on="Cluster 15" class="Clust (strict)"("Visible"=w316) -> ()  [unwired: 2 in, 2 out]
            n437 = property on="Cluster 13" class="Clust (strict)"("Visible"=TRUE) -> ()  [unwired: 2 in, 2 out]
            n438 = property on="Cluster 18" class="Clust (strict)"("Visible"=w316) -> ()  [unwired: 2 in, 2 out]
            n439 = property on="Cluster 17" class="Clust (strict)"("Visible"=w316) -> ()  [unwired: 2 in, 2 out]
          }
          frame 4 {
            w319 = FALSE
            n440 = property on="Cluster 15" class="Clust (strict)"("Visible"=TRUE) -> ()  [unwired: 2 in, 2 out]
            n441 = property on="Cluster 14" class="Clust (strict)"("Visible"=w319) -> ()  [unwired: 2 in, 2 out]
            n442 = property on="Cluster 13" class="Clust (strict)"("Visible"=w319) -> ()  [unwired: 2 in, 2 out]
            n443 = property on="Cluster 16" class="Clust (strict)"("Visible"=w319) -> ()  [unwired: 2 in, 2 out]
            n444 = property on="Cluster 18" class="Clust (strict)"("Visible"=w319) -> ()  [unwired: 2 in, 2 out]
            n445 = property on="Cluster 17" class="Clust (strict)"("Visible"=w319) -> ()  [unwired: 2 in, 2 out]
          }
          frame 5 {
            w321 = FALSE
            n446 = property on="Cluster 15" class="Clust (strict)"("Visible"=w321) -> ()  [unwired: 2 in, 2 out]
            n447 = property on="Cluster 14" class="Clust (strict)"("Visible"=w321) -> ()  [unwired: 2 in, 2 out]
            n448 = property on="Cluster 17" class="Clust (strict)"("Visible"=w321) -> ()  [unwired: 2 in, 2 out]
            n449 = property on="Cluster 16" class="Clust (strict)"("Visible"=TRUE) -> ()  [unwired: 2 in, 2 out]
            n450 = property on="Cluster 18" class="Clust (strict)"("Visible"=w321) -> ()  [unwired: 2 in, 2 out]
            n451 = property on="Cluster 13" class="Clust (strict)"("Visible"=w321) -> ()  [unwired: 2 in, 2 out]
          }
          frame 6 {
            w323 = FALSE
            n452 = property on="Cluster 15" class="Clust (strict)"("Visible"=w323) -> ()  [unwired: 2 in, 2 out]
            n453 = property on="Cluster 16" class="Clust (strict)"("Visible"=w323) -> ()  [unwired: 2 in, 2 out]
            n454 = property on="Cluster 18" class="Clust (strict)"("Visible"=w323) -> ()  [unwired: 2 in, 2 out]
            n455 = property on="Cluster 14" class="Clust (strict)"("Visible"=TRUE) -> ()  [unwired: 2 in, 2 out]
            n456 = property on="Cluster 13" class="Clust (strict)"("Visible"=w323) -> ()  [unwired: 2 in, 2 out]
            n457 = property on="Cluster 17" class="Clust (strict)"("Visible"=w323) -> ()  [unwired: 2 in, 2 out]
          }
        }
        n458 = case shown="6" w288 {
          frame 1, Default {
            w300 = FALSE
            n459 = property on="Cluster 22" class="Clust (strict)"("Visible"=w300) -> ()  [unwired: 2 in, 2 out]
            n460 = property on="Cluster 19" class="Clust (strict)"("Visible"=TRUE) -> ()  [unwired: 2 in, 2 out]
            n461 = property on="Cluster 20" class="Clust (strict)"("Visible"=w300) -> ()  [unwired: 2 in, 2 out]
            n462 = property on="Cluster 21" class="Clust (strict)"("Visible"=w300) -> ()  [unwired: 2 in, 2 out]
            n463 = property on="Cluster 23" class="Clust (strict)"("Visible"=w300) -> ()  [unwired: 2 in, 2 out]
            n464 = property on="Cluster 24" class="Clust (strict)"("Visible"=w300) -> ()  [unwired: 2 in, 2 out]
          }
          frame 2 {
            w302 = FALSE
            n465 = property on="Cluster 22" class="Clust (strict)"("Visible"=w302) -> ()  [unwired: 2 in, 2 out]
            n466 = property on="Cluster 21" class="Clust (strict)"("Visible"=w302) -> ()  [unwired: 2 in, 2 out]
            n467 = property on="Cluster 20" class="Clust (strict)"("Visible"=TRUE) -> ()  [unwired: 2 in, 2 out]
            n468 = property on="Cluster 19" class="Clust (strict)"("Visible"=w302) -> ()  [unwired: 2 in, 2 out]
            n469 = property on="Cluster 23" class="Clust (strict)"("Visible"=w302) -> ()  [unwired: 2 in, 2 out]
            n470 = property on="Cluster 24" class="Clust (strict)"("Visible"=w302) -> ()  [unwired: 2 in, 2 out]
          }
          frame 3 {
            w305 = FALSE
            n471 = property on="Cluster 22" class="Clust (strict)"("Visible"=w305) -> ()  [unwired: 2 in, 2 out]
            n472 = property on="Cluster 20" class="Clust (strict)"("Visible"=w305) -> ()  [unwired: 2 in, 2 out]
            n473 = property on="Cluster 19" class="Clust (strict)"("Visible"=w305) -> ()  [unwired: 2 in, 2 out]
            n474 = property on="Cluster 21" class="Clust (strict)"("Visible"=TRUE) -> ()  [unwired: 2 in, 2 out]
            n475 = property on="Cluster 23" class="Clust (strict)"("Visible"=w305) -> ()  [unwired: 2 in, 2 out]
            n476 = property on="Cluster 24" class="Clust (strict)"("Visible"=w305) -> ()  [unwired: 2 in, 2 out]
          }
          frame 4 {
            w306 = FALSE
            n477 = property on="Cluster 20" class="Clust (strict)"("Visible"=w306) -> ()  [unwired: 2 in, 2 out]
            n478 = property on="Cluster 21" class="Clust (strict)"("Visible"=w306) -> ()  [unwired: 2 in, 2 out]
            n479 = property on="Cluster 19" class="Clust (strict)"("Visible"=w306) -> ()  [unwired: 2 in, 2 out]
            n480 = property on="Cluster 23" class="Clust (strict)"("Visible"=TRUE) -> ()  [unwired: 2 in, 2 out]
            n481 = property on="Cluster 22" class="Clust (strict)"("Visible"=w306) -> ()  [unwired: 2 in, 2 out]
            n482 = property on="Cluster 24" class="Clust (strict)"("Visible"=w306) -> ()  [unwired: 2 in, 2 out]
          }
          frame 5 {
            w308 = FALSE
            n483 = property on="Cluster 22" class="Clust (strict)"("Visible"=w308) -> ()  [unwired: 2 in, 2 out]
            n484 = property on="Cluster 20" class="Clust (strict)"("Visible"=w308) -> ()  [unwired: 2 in, 2 out]
            n485 = property on="Cluster 21" class="Clust (strict)"("Visible"=w308) -> ()  [unwired: 2 in, 2 out]
            n486 = property on="Cluster 24" class="Clust (strict)"("Visible"=TRUE) -> ()  [unwired: 2 in, 2 out]
            n487 = property on="Cluster 23" class="Clust (strict)"("Visible"=w308) -> ()  [unwired: 2 in, 2 out]
            n488 = property on="Cluster 19" class="Clust (strict)"("Visible"=w308) -> ()  [unwired: 2 in, 2 out]
          }
          frame 6 {
            w311 = FALSE
            n489 = property on="Cluster 20" class="Clust (strict)"("Visible"=w311) -> ()  [unwired: 2 in, 2 out]
            n490 = property on="Cluster 21" class="Clust (strict)"("Visible"=w311) -> ()  [unwired: 2 in, 2 out]
            n491 = property on="Cluster 24" class="Clust (strict)"("Visible"=w311) -> ()  [unwired: 2 in, 2 out]
            n492 = property on="Cluster 22" class="Clust (strict)"("Visible"=TRUE) -> ()  [unwired: 2 in, 2 out]
            n493 = property on="Cluster 19" class="Clust (strict)"("Visible"=w311) -> ()  [unwired: 2 in, 2 out]
            n494 = property on="Cluster 23" class="Clust (strict)"("Visible"=w311) -> ()  [unwired: 2 in, 2 out]
          }
        }
      }
      frame "init" {
        w357 = T8."Disabled and Grayed Out" ("Disabled")
        w359 = i32[] [0, 0, 0, 0] ("我家骰子點數")
        w360 = 0
        w361 = FALSE
        w363 = i32[] [0, 0, 0, 0] ("我家骰子點數")
        w362 = 0
        n495 = global read "global variable-賭金金額.vi" "賭金金額"() -> (→"賭金金額":i32)
        n496 = property on="遊戲開始" class="Bool"("DisabledEnum"=T8."Enabled" ("Disabled")) -> ()  [unwired: 2 in, 2 out]
        n497 = One Button Dialog(message="歡迎遊玩十八仔，在開始遊戲之前請先詳細閱讀左邊的遊戲說明") -> ()  [unwired: 1 in, 1 out]
        n498 = property on="停止擲骰子" class="Bool"("DisabledEnum"=w357) -> ()  [unwired: 2 in, 2 out]
        n499 = property on="進入下一輪" class="Bool"("DisabledEnum"=w357) -> ()  [unwired: 2 in, 2 out]
        "此輪賺取/賠掉金額" <- w362
        "經歷輪數" <- w362
        "總共賺取/賠掉金額" <- w362
        "莊家重複累加器" <- w362
        "莊家骰子點數" <- w363
        "玩家骰子點數" <- w363
        "玩家重複累加器" <- w362
        "玩家是否是一色" <- w361
        "莊家是否是一色" <- w361
        "莊家所得點數" <- w360
        "玩家所得點數" <- w360
        "莊家計算點數之兩顆骰子" <- w359
        "玩家計算點數之兩顆骰子" <- w359
      }
    }
    n500 = Equal?(x="退出遊戲", y=TRUE) -> (x = y?=w5:bool)
    n501 = case shown="True" w5 {
      tunnel: "退出遊戲" -> [w9 w11]
      tunnel: [w9 w11] -> w4
      frame False {
      }
      frame True {
        n502 = local read "賭金金額"() -> (w10:i32)
        n503 = global write "global variable-賭金回傳.vi" "賭金回傳"(w10) -> ()
      }
    }
  }
  "Enum" <- enum16{"otherside", "myside"}."otherside" ("Enum")
